vi "Delete_SoundFile.vi"(8 "error in (no error)":errorcluster, 11 "File Path In":path) -> (0 "error out":errorcluster)   [LabVIEW 2018, in "MerriamWebsterJSON.lvlib"]
uses:
  MerriamWebsterJSON.lvlib
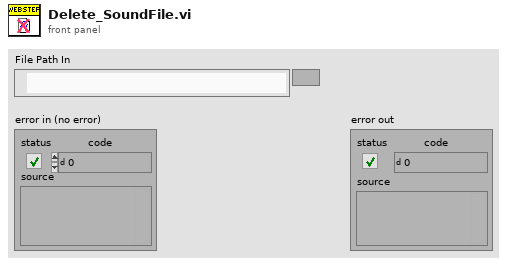
[diagram p1: front panel]
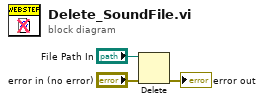
[diagram p0: block diagram]
diagram:
  n1 = Delete(path (use dialog)="File Path In", error in="error in (no error)") -> (error out=→"error out":errorcluster)  [unwired: 3 in, 2 out]
